vi "OPC_Tag_PLC_Tag_Generator.vi"(9 "Table Name":string, 10 "Columns":string[](array[string]), 11 "column information":T2(array[cluster])) -> (1 "OPC Tag only":string, 3 "OPC Tags":string, 4 "PLC Tag only":string, 5 "Header":string="Tag Name,Address,Data Type,Respect Data Type,Client Access,Scan Rate,Scaling,Raw Low,Raw High,Scaled Low,Scaled High,Scaled Data Type,Clamp Low,Clamp High,Eng Units,Description,Negate Value", 6 "PLC Header":string="Tag Name,Address,Data Type,Respect Data Type,Client Access,Scan Rate,Scaling,Raw Low,Raw High,Scaled Low,Scaled High,Scaled Data Type,Clamp Low,Clamp High,Eng Units,Description,Negate Value")   [LabVIEW 2020]
uses:
  <vilib>/addons/database/Auxilliary.llb/DB Tools DataTypes.ctl
  <userlib>/_OpenG.lib/array/array.llb/Search 1D Array (String)__ogtk.vi
  <userlib>/_OpenG.lib/array/array.llb/Delete Elements from 1D Array (String)__ogtk.vi
  <vilib>/regexp/Match Regular Expression.xnode
  <vilib>/addons/database/NI_Database_API.lvlib
panel:
  out "MACHINE NO":string
  out "Indices of Elements":i32[](array[numeric])
  out "column information 2":T2(array[cluster])
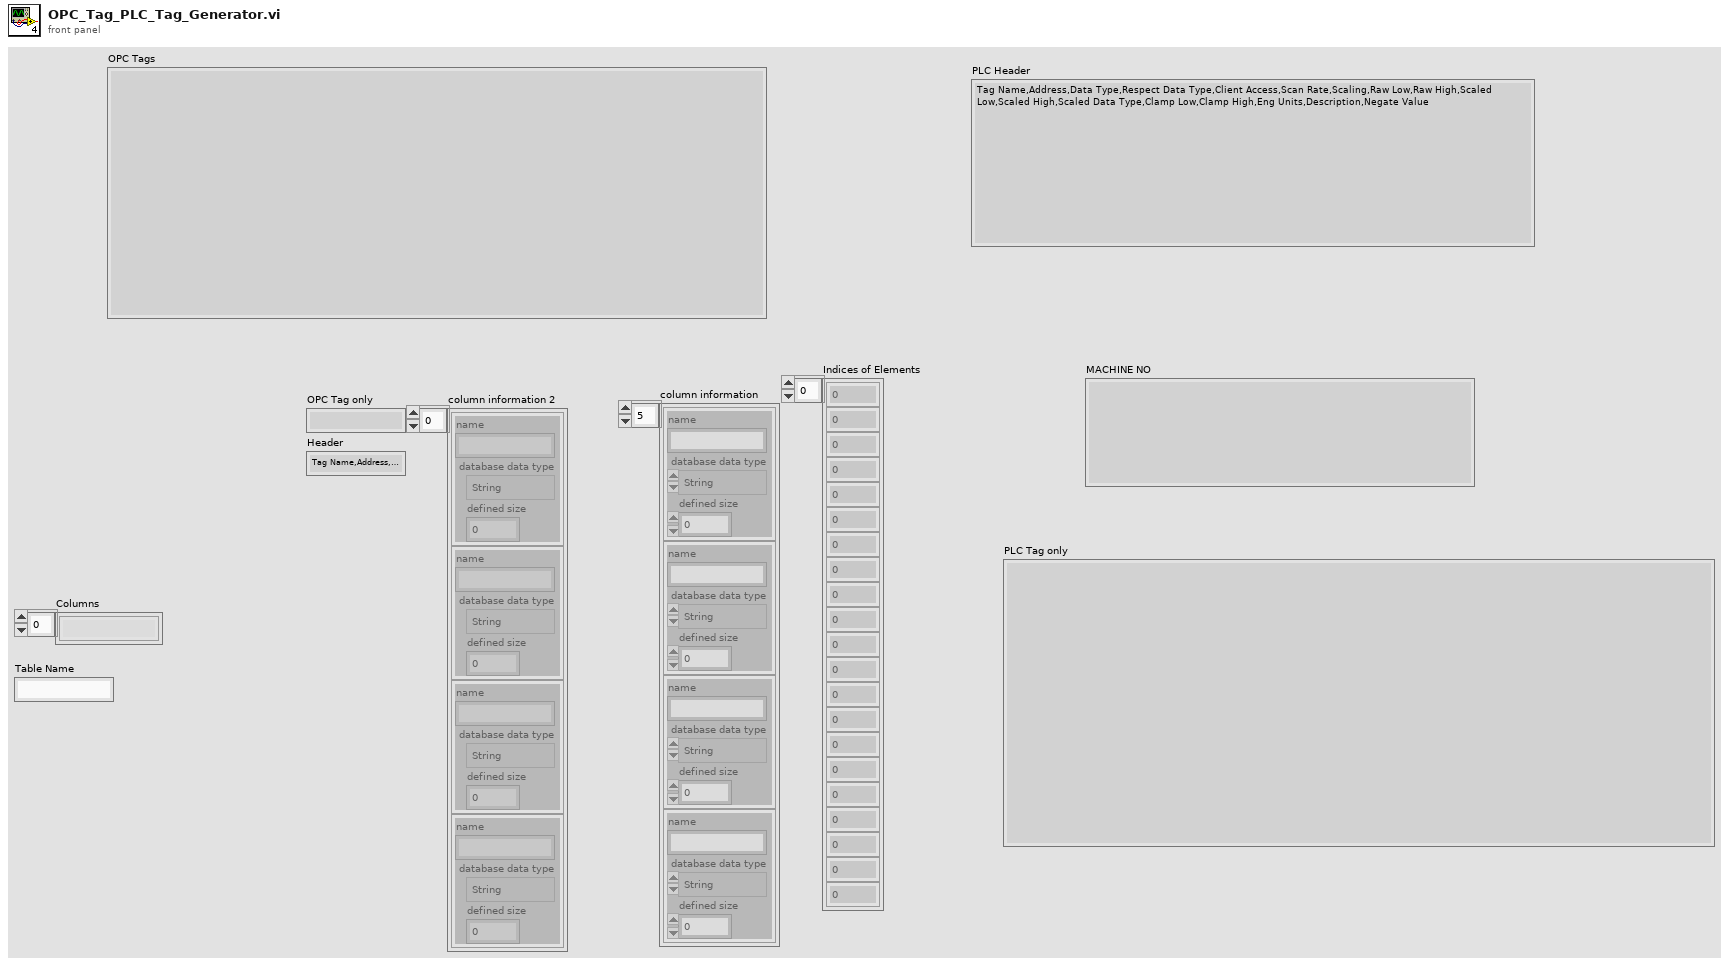
[diagram p1: front panel]
types:
  T1 = typedef "NI_Database_API.lvlib/DB Tools DataTypes.ctl" = enum16{"String", "Long (I32)", "Single (SGL)", "Double (DBL)", "Date/Time", "Binary"}
  T2 = cluster{"name":string, "database data type":T1, "defined size":i32}[]
  T3 = cluster{"name":string, "database data type":T1, "defined size":i32}
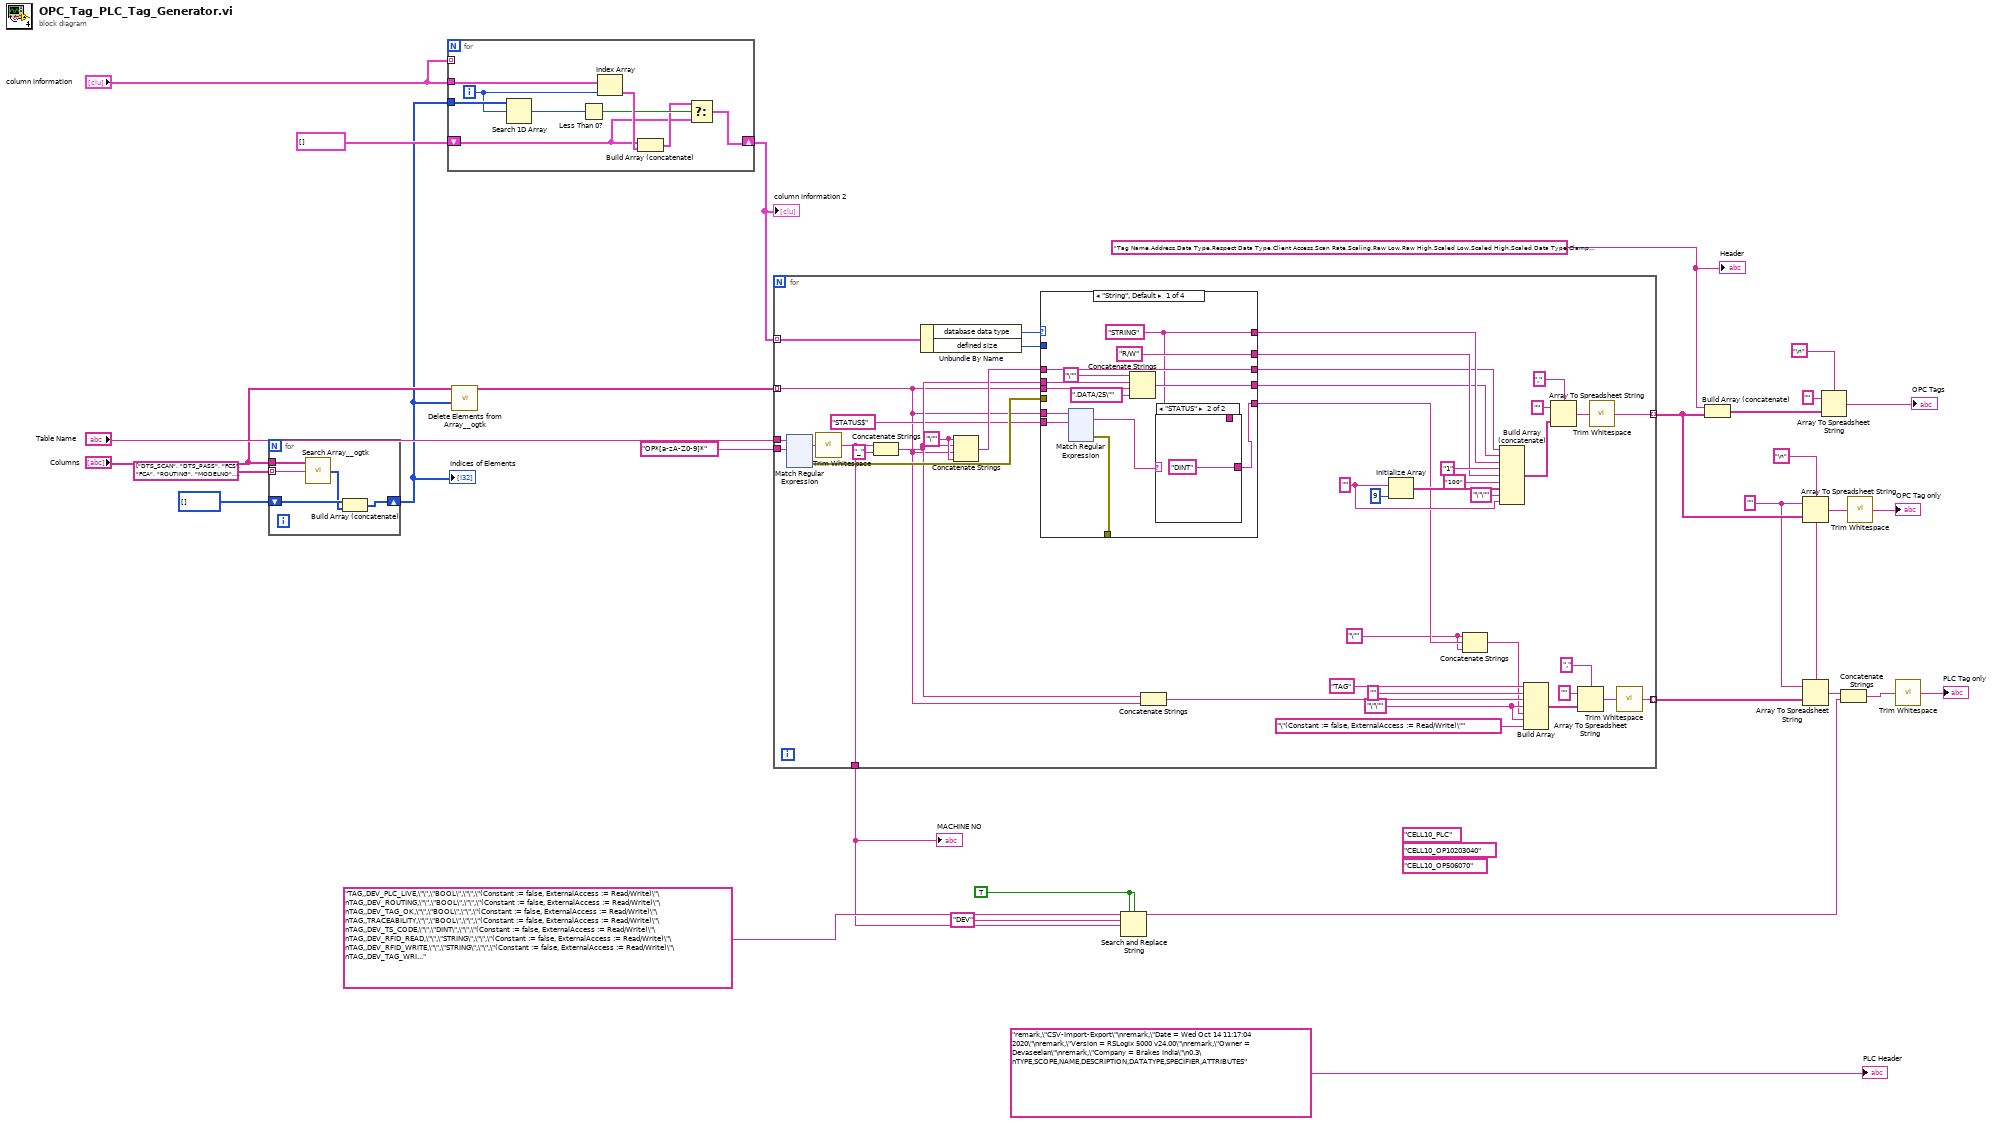
[diagram p0: block diagram]
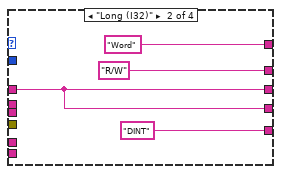
[diagram p3: hidden frame]
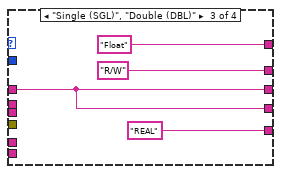
[diagram p4: hidden frame]
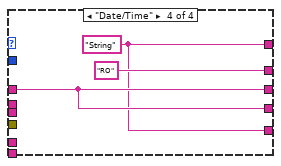
[diagram p5: hidden frame]
diagram:
  (unwired) "CELL10_OP506070" ("format string")
  (unwired) "CELL10_OP10203040" ("format string")
  (unwired) "CELL10_PLC" ("format string")
  w3 = TRUE ("replace all? (F)")
  w10 = "" ("format string")
  w9 = "\n" ("delimiter (Tab)")
  w28 = "Tag Name,Address,Data Type,Respect Data Type,Client Access,Scan Rate,Scaling,Raw Low,Raw High,Scaled Low,Scaled High,Scaled Data Type,Clamp Low,Clamp High,Eng Units,Description,Negate Value" ("String")
  n1 = for {
    tunnel: "Columns" -> [w35]
    tunnel: string[] ["DTS_SCAN", "DTS_PASS", "FCS", "FCA", "ROUTING", "MODELNO", "WORKORDER", "CELLNO", "PROFITCENTRE", "MACHINECODE", "OPERATIONCODE"] ("columns") -> [w34] mode=indexing
    shift-right: [w32] -> w14
    shift-left: i32[] [] ("Indices of Elements") -> [w33]
    n2 = call-poly <userlib>:"Search Array__ogtk.vi"("Array"=w35, "Element Data"=w34) -> ("Indices of Elements"=w31:i32[])  [unwired: 7 in]
    n3 = Build Array (concatenate)(w33, w31) -> (w32:i32[])
  }
  "Indices of Elements" <- w14
  n4 = for {
    tunnel: "column information" -> [w44]
    shift-right: [w39] -> w21
    shift-left: T2 [] ("column information") -> [w40]
    tunnel: w14 -> [w38]
    tunnel: "column information" -> [_] mode=indexing
    i -> [w37]
    n5 = Search 1D Array(1D array=w38, element=w37) -> (index of element=w36:i32)  [unwired: 1 in]
    n6 = Less Than 0?(x=w36) -> (x < 0?=w42:bool)
    n7 = Index Array(array=w44, index=w37) -> (element=w43:T3)
    n8 = Build Array (concatenate)(w40, w43) -> (w41:T2)
    n9 = Select(t=w41, s=w42, f=w40) -> (s? t:f=w39:T2)
  }
  "column information 2" <- w21
  n10 = call-poly <userlib>:"Delete Elements from Array__ogtk.vi"("indices"=w14, "array"="Columns") -> ("array w/ subset deleted"=w19:string[])  [unwired: 8 in, 1 out]
  n11 = for {
    tunnel: w21 -> [w86] mode=indexing
    tunnel: "OP*[a-zA-Z0-9]*" ("String") -> [w84]
    tunnel: [w74] -> w18 mode=indexing
    tunnel: w19 -> [w45] mode=indexing
    tunnel: "Table Name" -> [w65]
    tunnel: [w54] -> w11 mode=indexing
    tunnel: [w49] -> w4
    w51 = "\"" ("string")
    w53 = "\"\"" ("format string")
    w70 = ""
    w63 = "\"" ("string")
    n12 = xnode "Match Regular Expression"("input string"=w65, "regular expression"=w84) -> ("whole match"=w66:string, "error out"=w64:errorcluster)  [unwired: 4 in, 3 out]
    n13 = call <vilib>:"Trim Whitespace.vi"("string"=w66) -> ("trimmed string"=w49:string)  [unwired: 1 in]
    n14 = Concatenate Strings(w49, "_" ("string")) -> (w47:string)
    n15 = Unbundle By Name(w86) -> ("database data type"=w83:T1, "defined size"=w85:i32)
    n16 = Concatenate Strings(w63, w47, w45, w63) -> (w69:string)
    n17 = case shown="\"String\", Default" w83 {
      tunnel: w85 -> [_ _ _ _]
      tunnel: w64 -> [_ _ _ _]
      tunnel: [w201 "Word" "Float" w338] -> w82
      tunnel: ["R/W" "R/W" "R/W" "RO"] -> w80
      tunnel: w69 -> [w212 w331 w335 w339]
      tunnel: [w212 w331 w335 w339] -> w68
      tunnel: w45 -> [w211 _ _ _]
      tunnel: [w209 w331 w335 w339] -> w67
      tunnel: w47 -> [w207 _ _ _]
      tunnel: [w202 "DINT" "REAL" w338] -> w52
      tunnel: w45 -> [w206 _ _ _]
      tunnel: "STATUS$" -> [w205 _ _ _]
      tunnel: [w204 _ _ _] -> _
      frame "String", Default {
        w201 = "STRING"
        n18 = xnode "Match Regular Expression"("input string"=w206, "regular expression"=w205) -> ("whole match"=w203:string, "error out"=w204:errorcluster)  [unwired: 4 in, 3 out]
        n19 = Concatenate Strings("\"" ("string"), w207, w211, ".DATA/25\"" ("string")) -> (w209:string)
        n20 = case shown="\"STATUS\"" w203 {
          tunnel: [w214 "DINT"] -> w202
          tunnel: w201 -> [w214 _]
          frame "False", Default {
          }
          frame "STATUS" {
          }
        }
      }
      frame "Long (I32)" {
      }
      frame "Single (SGL)", "Double (DBL)" {
      }
      frame "Date/Time" {
        w338 = "String"
      }
    }
    n21 = Concatenate Strings(w47, w45) -> (w61:string)
    n22 = Initialize Array(w70, 9 ("dimension size")) -> (w72:string[])
    n23 = Concatenate Strings(w51, w52, w51) -> (w50:string)
    n24 = Build Array (concatenate)(w68, w67, w82, "1", w80, "100" ("element"), w72, "\"\"" ("element"), w70) -> (w77:string[])
    n25 = Build Array("TAG" ("format string"), "" ("format string"), w61, w53, w50, w53, "\"(Constant := false, ExternalAccess := Read/Write)\"" ("format string")) -> (w55:string[])
    n26 = Array To Spreadsheet String(delimiter (Tab)=",", array=w77, 3:"" ("format string")) -> (spreadsheet string=w75:string)
    n27 = Array To Spreadsheet String(delimiter (Tab)=",", array=w55, 3:"" ("format string")) -> (spreadsheet string=w58:string)
    n28 = call <vilib>:"Trim Whitespace.vi"("string"=w75) -> ("trimmed string"=w74:string)  [unwired: 1 in]
    n29 = call <vilib>:"Trim Whitespace.vi"("string"=w58) -> ("trimmed string"=w54:string)  [unwired: 1 in]
  }
  "MACHINE NO" <- w4
  n30 = Search and Replace String(replace all?=w3, case sensitive?=w3, input string="TAG,,DEV_PLC_LIVE,\"\",\"BOOL\",\"\",\"(Constant := false, ExternalAccess := Read/Write)\"\nTAG,,DEV_ROUTING,\"\",\"BOOL\",\"\",\"(Constant := false, ExternalAccess := Read/Write)\"\nTAG,,DEV_TAG_OK,\"\",\"BOOL\",\"\",\"(Constant := false, ExternalAccess := Read/Write)\"\nTAG,,TRACEABILITY,\"\",\"BOOL\",\"\",\"(Constant := false, ExternalAccess := Read/Write)\"\nTAG,,DEV_TS_CODE,\"\",\"DINT\",\"\",\"(Constant := false, ExternalAccess := Read/Write)\"\nTAG,,DEV_RFID_READ,\"\",\"STRING\",\"\",\"(Constant := false, ExternalAccess := Read/Write)\"\nTAG,,DEV_RFID_WRITE,\"\",\"STRING\",\"\",\"(Constant := false, ExternalAccess := Read/Write)\"\nTAG,,DEV_TAG_WRITE,\"\",\"BOOL\",\"\",\"(Constant := false, ExternalAccess := Read/Write)\"" ("delimiter (Tab)"), search string="DEV", replace string=w4) -> (result string=w1:string)  [unwired: 3 in, 3 out]
  n31 = Build Array (concatenate)(w28, w18) -> (w27:string[])
  n32 = Array To Spreadsheet String(delimiter (Tab)=w9, array=w18, 3:w10) -> (spreadsheet string=w17:string)
  n33 = Array To Spreadsheet String(delimiter (Tab)=w9, array=w11, 3:w10) -> (spreadsheet string=w7:string)
  n34 = Array To Spreadsheet String(delimiter (Tab)="\n", array=w27, 3:"" ("format string")) -> (spreadsheet string=→"OPC Tags":string)
  n35 = Concatenate Strings(w7, w1) -> (w2:string)
  n36 = call <vilib>:"Trim Whitespace.vi"("string"=w17) -> ("trimmed string"=→"OPC Tag only":string)  [unwired: 1 in]
  n37 = call <vilib>:"Trim Whitespace.vi"("string"=w2) -> ("trimmed string"=→"PLC Tag only":string)  [unwired: 1 in]
  "Header" <- w28
  "PLC Header" <- "remark,\"CSV-Import-Export\"\nremark,\"Date = Wed Oct 14 11:17:04 2020\"\nremark,\"Version = RSLogix 5000 v24.00\"\nremark,\"Owner = Devaseelan\"\nremark,\"Company = Brakes India\"\n0.3\nTYPE,SCOPE,NAME,DESCRIPTION,DATATYPE,SPECIFIER,ATTRIBUTES" ("String")
